vi "String to Number.vi"(0 "Data":string, 7 "Expression":string) -> (8 "Number":i32)   [LabVIEW 2010]
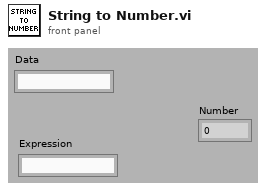
[diagram p1: front panel]
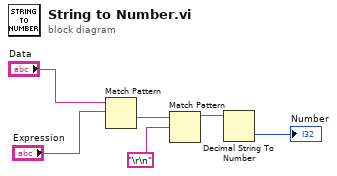
[diagram p0: block diagram]
diagram:
  n1 = Match Pattern(string="Data", regular expression="Expression") -> (after substring=w4:string)  [unwired: 1 in, 3 out]
  n2 = Match Pattern(string=w4, regular expression="\r\n") -> (before substring=w2:string)  [unwired: 1 in, 3 out]
  n3 = Decimal String To Number(string=w2) -> (number=→"Number":i32)  [unwired: 2 in, 1 out]
